vi "Method.vi"(4 "Value":refnum<class "Abs_I32 Integer.lvclass">) -> (1 "Result":refnum<class "Abs_Boolean.lvclass">)   [LabVIEW 2021, in "Equal 0_I32.lvclass"]
uses:
  Equal 0_I32.lvclass
  Abs_Types/I32 Integer/Abs_I32 Integer.lvclass
  Abs_Types/Boolean/Abs_Boolean.lvclass
  C:/TSA/LV_Abstract/Source/Functions/Support/Compare/One Term/I32/AbsComp_One Term_I32.lvclass
  C:/Program Files (x86)/National Instruments/LabVIEW 2021/vi.lib/TSA/Abstract Data Classes/Abs_Types/Boolean/Abs_Boolean.lvclass
  Support/Compare/One Term/I32/AbsComp_One Term_I32.lvclass/AbsComp_One Term_I32.ctl
  Support/Compare/One Term/I32/Properties/Write Numeric A.vi
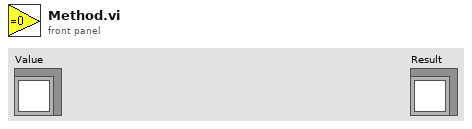
[diagram p1: front panel]
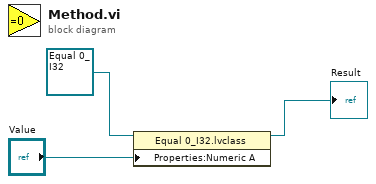
[diagram p0: block diagram]
diagram:
  n1 = property class="Equal 0_I32.lvclass"(reference=refnum<class "Equal 0_I32.lvclass"> refnum ("Greater 0_U64.lvclass"), "Properties:Numeric A"="Value") -> (reference out=→"Result":refnum<class "Equal 0_I32.lvclass">)  [unwired: 1 in, 1 out]
